vi "Send Message.vi"(0 "reference in":refnum<class "Generic Utilities.lvclass">, 5 "error in (no error)":errorcluster, 6 "Ignore Cursor":bool, 7 "Message (\"\" closes the window)":string, 9 "Make Cursor Busy?":bool) -> (14 "reference out":refnum<class "Generic Utilities.lvclass">, 19 "error out":errorcluster)   [LabVIEW 2020, in "Generic Utilities.lvclass"]
uses:
  Generic Utilities.lvclass
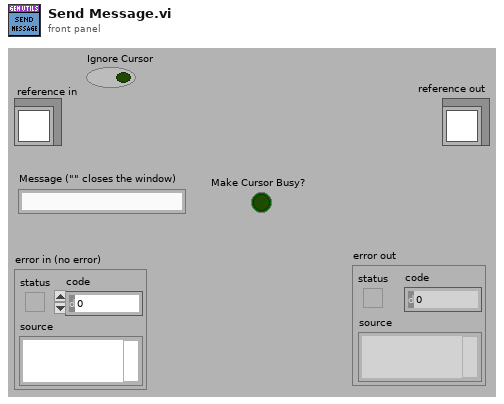
[diagram p1: front panel]
types:
  T1 = enum32{"Invalid", "Standard", "Closed", "Hidden", "Minimized", "Maximized"}
  T2 = typedef "Generic Utilities.lvclass/ObjectAttributes.ctl" = cluster{"GUI Parameters":T3, "State Machine Control":cluster{"Timeout":i32, "State Queue":string[], "State History":string[], "State History Length":i32}, "Logging File Path":path, "OBJ not a refnum?":bool, "Timer Start":timestamp, "FP Refnums":T4}
  T3 = typedef "Generic Utilities.lvclass/GUI Parameters.ctl" = cluster{"Application Name":string, "GUI VI Ref":refnum<vi>, "Close Panel?":bool, "Message Window ref":refnum<vi>, "Version #":string}
  T4 = typedef "Generic Utilities.lvclass/FP Refnums.ctl" = cluster{"Panel refnum":refnum<vi>, "Control Labels":string[], "Refnums":refnum<vi>[]}
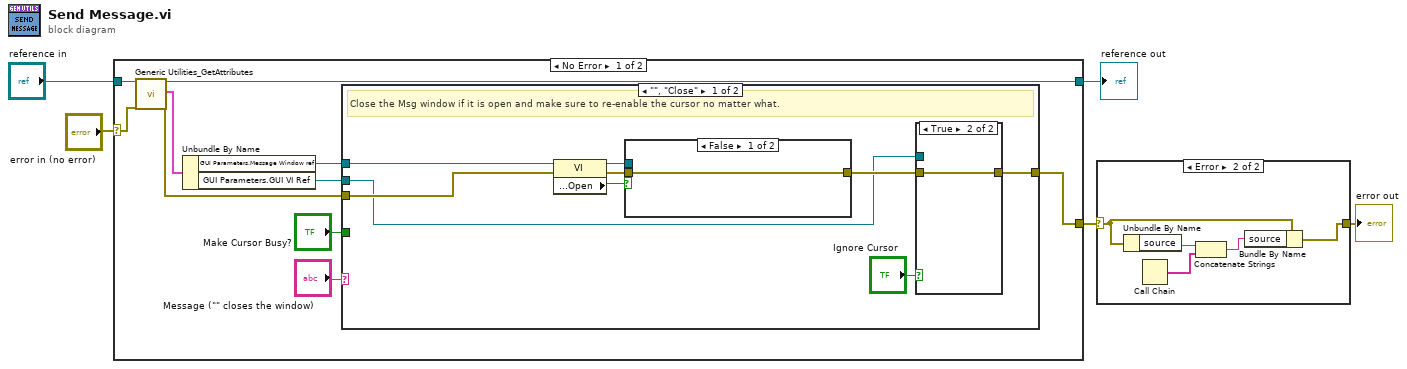
[diagram p0: block diagram]
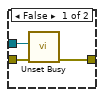
[diagram p3: hidden frame]
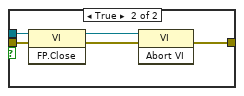
[diagram p4: hidden frame]
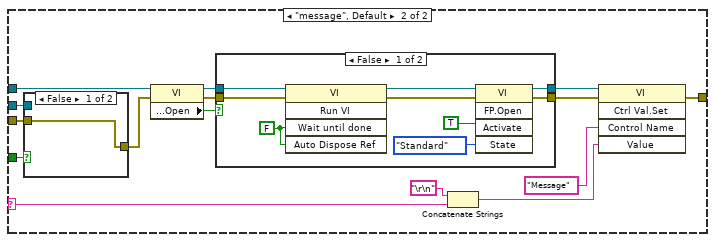
[diagram p5: hidden frame]
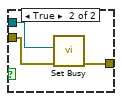
[diagram p6: hidden frame]
diagram:
  n1 = case shown="No Error" "error in (no error)" {
    selector: "error in (no error)" -> [w15 w66]
    tunnel: [w9 w66] -> w2
    tunnel: [w14 w65] -> w3
    tunnel: "reference in" -> [w12 w65]
    frame No Error {
      n2 = call "Generic Utilities_GetAttributes.vi"("reference in"=w12, "error in (no error)"=w15) -> ("reference out"=w14:refnum<class "Generic Utilities.lvclass">, "attributes"=w13:T2, "error out"=w10:errorcluster)  [unwired: 14 in, 1 out]
      n3 = Unbundle By Name(w13) -> ("GUI Parameters.Message Window ref"=w11:refnum<vi>, "GUI Parameters.GUI VI Ref"=w6:refnum<vi>)
      n4 = case shown="\"\", \"Close\"" "Message (\"\" closes the window)" {
        selector: "Message (\"\" closes the window)" -> [_ w39]
        tunnel: w11 -> [w21 w41]
        tunnel: w10 -> [w20 w37]
        tunnel: [w18 w40] -> w9
        tunnel: "Make Cursor Busy?" -> [_ w38]
        tunnel: w6 -> [w17 w35]
        frame "", "Close" {
          # "Close the Msg window if it is open and make sure to re-enable the cursor no matter what."
          n5 = property class="VI"(reference=w21, error in=w20) -> (reference out=w23:refnum<vi>, error out=w22:errorcluster, "Front Panel.Open"=w24:bool)
          n6 = case shown="False" w24 {
            tunnel: [w29 w30] -> w19
            tunnel: w22 -> [w29 w34]
            tunnel: w23 -> [_ w33]
            frame False {
            }
            frame True {
              n7 = invoke class="VI" method="FP.Close"(reference=w33, error in=w34) -> (reference out=w32:refnum<vi>, error out=w31:errorcluster)  [unwired: 1 in, 1 out]
              n8 = invoke class="VI" method="Abort VI"(reference=w32, error in=w31) -> (error out=w30:errorcluster)  [unwired: 1 in, 2 out]
            }
          }
          n9 = case shown="True" "Ignore Cursor" {
            tunnel: w19 -> [w27 w28]
            tunnel: [w26 w28] -> w18
            tunnel: w17 -> [w25 _]
            frame False {
              n10 = call <vilib>:"Unset Busy.vi"("error in (no error)"=w27, "VI reference (current VI)"=w25) -> ("error out"=w26:errorcluster)  [unwired: 9 in]
            }
            frame True {
            }
          }
        }
        frame "message", Default {
          n11 = case shown="False" w38 {
            tunnel: w37 -> [w50 w53]
            tunnel: [w50 w52] -> w36
            tunnel: w35 -> [_ w51]
            frame False {
            }
            frame True {
              n12 = call <vilib>:"Set Busy.vi"("error in (no error)"=w53, "VI reference (current VI)"=w51) -> ("error out"=w52:errorcluster)  [unwired: 8 in, 1 out]
            }
          }
          n13 = property class="VI"(reference=w41, error in=w36) -> (reference out=w48:refnum<vi>, error out=w49:errorcluster, "Front Panel.Open"=w47:bool)
          n14 = case shown="False" w47 {
            tunnel: [w60 w64] -> w45
            tunnel: w49 -> [w55 w64]
            tunnel: w48 -> [w57 w63]
            tunnel: [w59 w63] -> w46
            frame False {
              w58 = FALSE ("Wait Until Done")
              n15 = invoke class="VI" method="Run VI"(reference=w57, error in=w55, "Wait until done"=w58, "Auto Dispose Ref"=w58) -> (reference out=w56:refnum<vi>, error out=w54:errorcluster)  [unwired: 1 in, 3 out]
              n16 = invoke class="VI" method="FP.Open"(reference=w56, error in=w54, "Activate"=TRUE, "State"=T1."Standard") -> (reference out=w59:refnum<vi>, error out=w60:errorcluster)  [unwired: 1 in, 3 out]
            }
            frame True {
            }
          }
          n17 = Concatenate Strings("\r\n", w39) -> (w42:string)
          n18 = invoke class="VI" method="Ctrl Val.Set"(reference=w46, error in=w45, "Control Name"="Message", "Value"=w42) -> (error out=w40:errorcluster)  [unwired: 1 in, 4 out]
        }
      }
    }
    frame Error {
    }
  }
  "reference out" <- w3
  n19 = case shown="Error" w2 {
    selector: w2 -> [w67 w70]
    tunnel: [w67 w68] -> w1
    frame No Error {
    }
    frame Error {
      n20 = Unbundle By Name(w70) -> ("source"=w72:string)
      n21 = Call Chain() -> (call chain=w71:string[])
      n22 = Concatenate Strings(w72, w71) -> (w69:string)
      n23 = Bundle By Name(cluster=w70, "source"=w69) -> (w68:errorcluster)
    }
  }
  "error out" <- w1
